vi "Send Output Value (DBL).vi"(8 "error in (no error)":errorcluster, 9 "DBL Value":dbl, 10 "Name":string, 11 "Template Module in":refnum<class "Template Module.lvclass">) -> (0 "error out":errorcluster, 3 "Template Module out":refnum<class "Template Module.lvclass">)   [LabVIEW 2018, in "Template Module.lvclass"]
uses:
  Template Module.lvclass
  Instrument Actor Messages/Set Output Msg/Set Output Msg.lvclass
  C:/Program Files/National Instruments/LabVIEW 2018/vi.lib/ActorFramework/Message/Message.lvclass
  NHMFL_Core/Libraries/Utilities/Output Value/Output Value.lvclass
  C:/github/NHMFL_Core/Libraries/Instruments/Results/Acquired Result/Acquired Result.lvclass
  Instrument Actor Messages/Set Output Msg/Set Output Msg.lvclass/Set Output Msg.ctl
  Instrument Actor Messages/Set Output Msg/Write Output value.vi
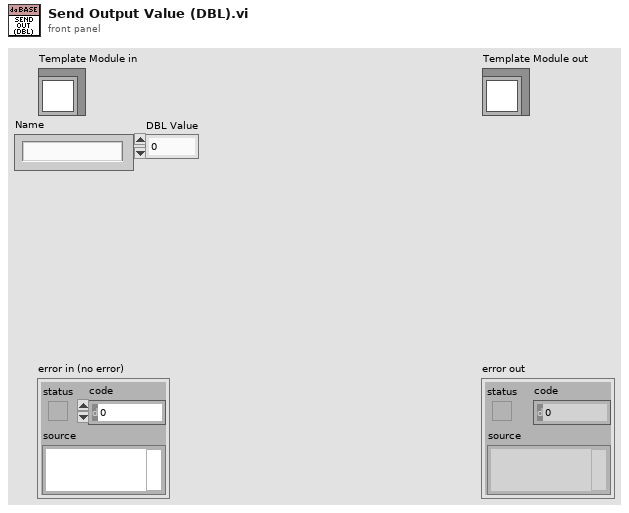
[diagram p1: front panel]
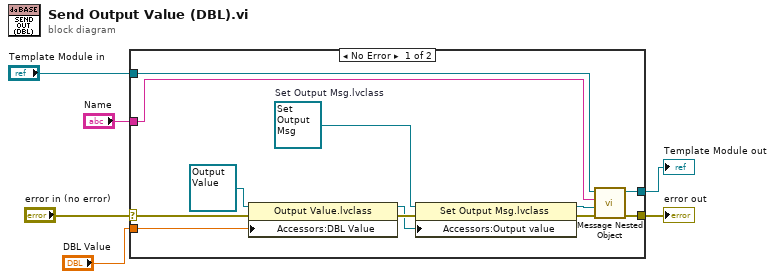
[diagram p0: block diagram]
diagram:
  n1 = case shown="No Error" "error in (no error)" {
    selector: "error in (no error)" -> [w9 w20]
    tunnel: [w7 w20] -> w5
    tunnel: [w8 w19] -> w3
    tunnel: "Template Module in" -> [w10 w19]
    tunnel: "DBL Value" -> [w12 _]
    tunnel: "Name" -> [w11 _]
    frame No Error {
      w13 = refnum<class "Set Output Msg.lvclass"> refnum  # Set Output Msg.lvclass
      n2 = property class="Output Value.lvclass"(reference=refnum<class "Output Value.lvclass"> refnum ("Output value"), error in=w9, "Accessors:DBL Value"=w12) -> (reference out=w15:refnum<class "Output Value.lvclass">, error out=w16:errorcluster)
      n3 = property class="Set Output Msg.lvclass"(reference=w13, error in=w16, "Accessors:Output value"=w15) -> (reference out=w17:refnum<class "Set Output Msg.lvclass">, error out=w18:errorcluster)
      n4 = call-dynamic "Message Nested Object.vi"("error in (no error)"=w18, "Message"=w17, "Name"=w11, "Application Controller in"=w10) -> ("error out"=w7:errorcluster, "Application Controller out"=w8:refnum<class "Template Module.lvclass">)  [unwired: 6 in]
    }
    frame Error {
    }
  }
  "error out" <- w5
  "Template Module out" <- w3
